vi "Usage3.vi"() -> ()   [LabVIEW 2017]
uses:
  Consumer/Abstract Consumer/Abstract Consumer.lvclass
  Message Queue/Message Queue/Message Queue.lvclass
  Message/Shutdown Message/Shutdown Message.lvclass
  SLSC Switch Consumer/SLSC Switch Consumer.lvclass
  Switch/Abstract Switch Init Parameters/Abstract Switch Init Parameters.lvclass
  Switch/Switch Connect Message/Switch Connect Message.lvclass
  Switch/Switch Disconnect All Message/Switch Disconnect All Message.lvclass
  Switch/Switch Disconnect Message/Switch Disconnect Message.lvclass
  Producer/Abstract Producer/Abstract Producer.lvclass
  Parameters/Abstract Init Parameters/Abstract Init Parameters.lvclass
  C:/azdo/jscholtz-message-queue-library/Source/Message Queue/Abstract Message Queue/Abstract Message Queue.lvclass
  C:/azdo/jscholtz-message-queue-library/Source/Switch/Abstract Switch Consumer/Abstract Switch Consumer.lvclass
  C:/azdo/jscholtz-message-queue-library/Source/Consumer/Abstract Consumer/Abstract Consumer.lvclass
  C:/azdo/jscholtz-message-queue-library/Source/Parameters/Abstract Init Parameters/Abstract Init Parameters.lvclass
  C:/azdo/jscholtz-message-queue-library/Source/Message/Abstract Request Message/Abstract Request Message.lvclass
  C:/azdo/jscholtz-message-queue-library/Source/Message/Abstract Message/Abstract Message.lvclass
panel:
  in  "Disconnect":bool
  in  "Disconnect All":bool
  in  "Connect":bool
  in  "Shutdown":bool
  out "error out":errorcluster
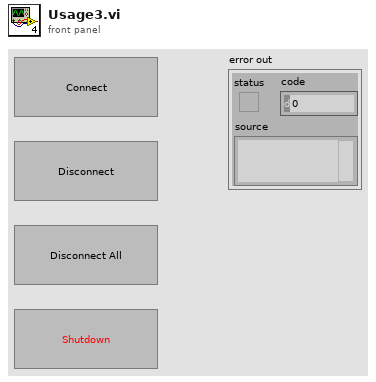
[diagram p1: front panel]
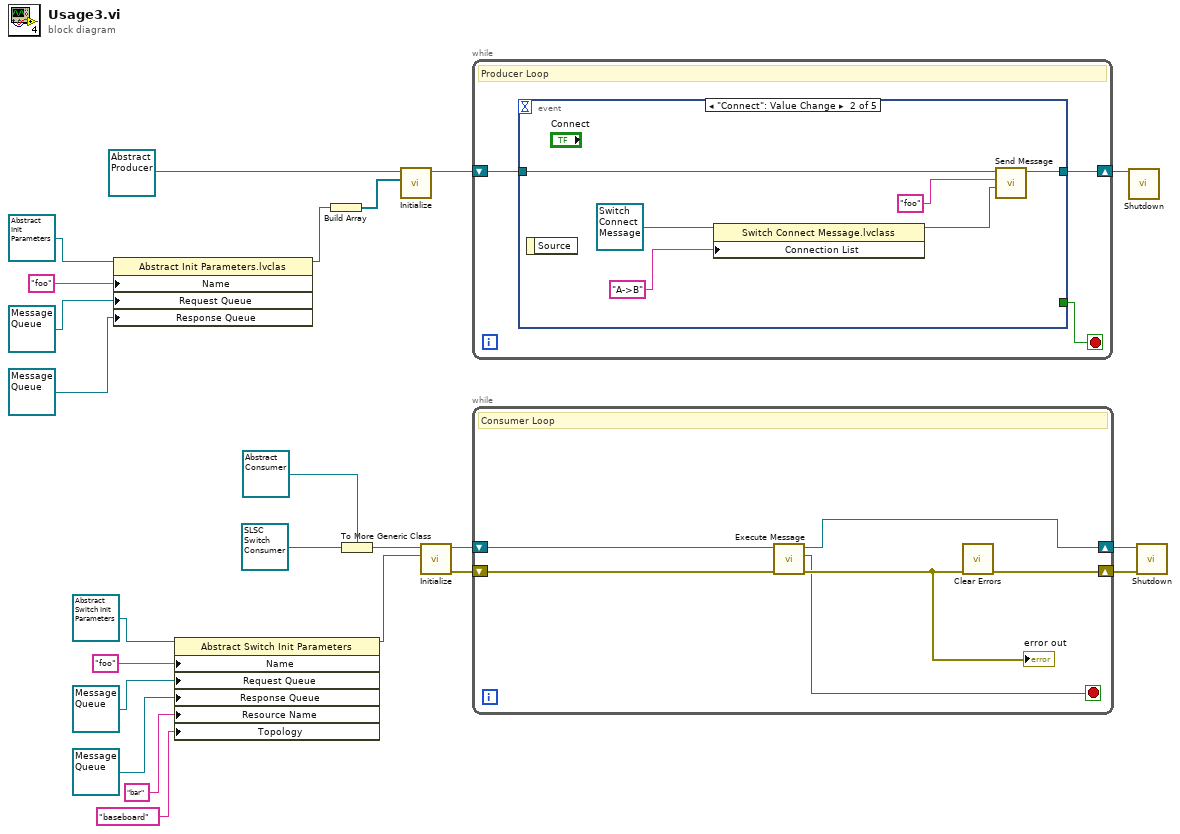
[diagram p0: block diagram]
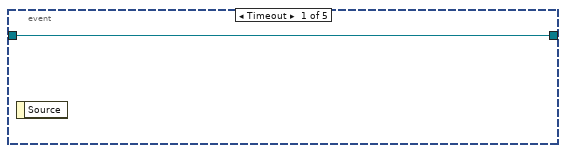
[diagram p2: hidden frame]
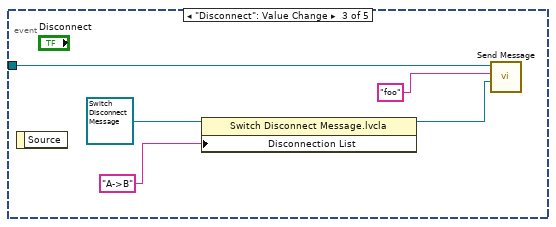
[diagram p3: hidden frame]
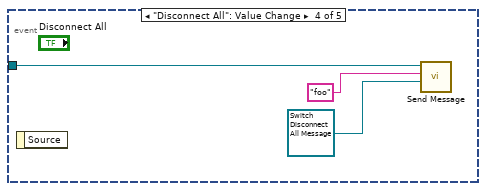
[diagram p4: hidden frame]
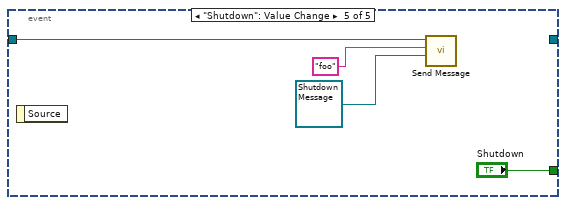
[diagram p5: hidden frame]
diagram:
  n1 = property class="Abstract Init Parameters.lvclas"(reference=refnum<class "Abstract Init Parameters.lvclass"> refnum ("Message Queue Library.lvlib:Abstract Init Parameters.lvclass"), "Name"="foo", "Request Queue"=refnum<class "Message Queue.lvclass"> refnum ("Message Queue Library.lvlib:Message Queue.lvclass"), "Response Queue"=refnum<class "Message Queue.lvclass"> refnum ("Message Queue Library.lvlib:Message Queue.lvclass")) -> (reference out=w3:refnum<class "Abstract Init Parameters.lvclass">)  [unwired: 1 in, 1 out]
  n2 = property class="Abstract Switch Init Parameters"(reference=refnum<class "Abstract Switch Init Parameters.lvclass"> refnum ("Message Queue Library.lvlib:Abstract Switch Init Parameters.lvclass"), "Name"="foo", "Request Queue"=refnum<class "Message Queue.lvclass"> refnum ("Message Queue Library.lvlib:Message Queue.lvclass"), "Response Queue"=refnum<class "Message Queue.lvclass"> refnum ("Message Queue Library.lvlib:Message Queue.lvclass"), "Resource Name"="bar", "Topology"="baseboard") -> (reference out=w18:refnum<class "Abstract Switch Init Parameters.lvclass">)  [unwired: 1 in, 1 out]
  n3 = Build Array(w3) -> (w8:refnum<class "Abstract Init Parameters.lvclass">[])
  n4 = To More Generic Class(target class=refnum<class "Abstract Consumer.lvclass"> refnum ("Abstract Consumer in"), reference=refnum<class "SLSC Switch Consumer.lvclass"> refnum ("Message Queue Library.lvlib:SLSC Switch Consumer.lvclass")) -> (generic class reference=w10:refnum<class "Abstract Consumer.lvclass">)
  n5 = call-dynamic "Initialize.vi"("Parameters in"=w8, "Abstract Producer in"=refnum<class "Abstract Producer.lvclass"> refnum ("Message Queue Library.lvlib:Abstract Producer.lvclass")) -> ("Abstract Producer out"=w2:refnum<class "Abstract Producer.lvclass">)  [unwired: 8 in, 1 out]
  n6 = call-dynamic "Initialize.vi"("Parameters in"=w18, "Abstract Consumer in"=w10) -> ("error out"=w23:errorcluster, "Abstract Consumer out"=w17:refnum<class "Abstract Consumer.lvclass">)  [unwired: 8 in]
  n7 = while {
    shift-right: [w24] -> w1
    shift-left: w2 -> [w25]
    stop <- w26 stop-if-true
    # "Producer Loop"
    n8 = event shown="[1] \"Connect\": Value Change" {
      selector: _ -> [_ _ _ _ _]
      dyn-events: _ -> [_ _ _ _ _]
      timeout: _ -> [_ _ _ _ _]
      tunnel: [_ _ _ _ "Shutdown"] -> w26
      tunnel: w25 -> [w27 w31 w35 w40 w43]
      tunnel: [w27 w28 _ _ _] -> w24
      event Timeout {
        n9 = event-data() -> ()  [unwired: 1 in, 1 out]
      }
      event "Connect": Value Change {
        n10 = event-data() -> ()  [unwired: 1 in, 1 out]
        n11 = property class="Switch Connect Message.lvclass"(reference=refnum<class "Switch Connect Message.lvclass"> refnum ("Message Queue Library.lvlib:Switch Connect Message.lvclass"), "Connection List"="A->B") -> (reference out=w30:refnum<class "Switch Connect Message.lvclass">)  [unwired: 1 in, 1 out]
        n12 = call-dynamic "Send Message.vi"("Message in"=w30, "Consumer in"="foo" ("Name"), "Abstract Producer in"=w31) -> ("Abstract Producer out"=w28:refnum<class "Abstract Producer.lvclass">)  [unwired: 6 in, 2 out]
      }
      event "Disconnect": Value Change {
        n13 = event-data() -> ()  [unwired: 1 in, 1 out]
        n14 = property class="Switch Disconnect Message.lvcla"(reference=refnum<class "Switch Disconnect Message.lvclass"> refnum ("Message Queue Library.lvlib:Switch Disconnect Message.lvclass"), "Disconnection List"="A->B" ("Connection List")) -> (reference out=w34:refnum<class "Switch Disconnect Message.lvclass">)  [unwired: 1 in, 1 out]
        n15 = call-dynamic "Send Message.vi"("Message in"=w34, "Consumer in"="foo" ("Name"), "Abstract Producer in"=w35) -> ()  [unwired: 6 in, 3 out]
      }
      event "Disconnect All": Value Change {
        n16 = event-data() -> ()  [unwired: 1 in, 1 out]
        n17 = call-dynamic "Send Message.vi"("Message in"=refnum<class "Switch Disconnect All Message.lvclass"> refnum ("Message Queue Library.lvlib:Switch Disconnect All Message.lvclass"), "Consumer in"="foo" ("Name"), "Abstract Producer in"=w40) -> ()  [unwired: 6 in, 3 out]
      }
      event "Shutdown": Value Change {
        n18 = event-data() -> ()  [unwired: 1 in, 1 out]
        n19 = call-dynamic "Send Message.vi"("Message in"=refnum<class "Shutdown Message.lvclass"> refnum ("Message Queue Library.lvlib:Shutdown Message.lvclass"), "Consumer in"="foo" ("Name"), "Abstract Producer in"=w43) -> ()  [unwired: 6 in, 3 out]
      }
    }
  }
  n20 = while {
    shift-right: [w46] -> w14
    shift-left: w23 -> [w51]
    shift-right: [w47] -> w13
    shift-left: w17 -> [w48]
    stop <- w49 stop-if-true
    # "Consumer Loop"
    n21 = call "Execute Message.vi"("error in (no error)"=w51, "Abstract Consumer in"=w48) -> ("error out"=w50:errorcluster, "Stop?"=w49:bool, "Abstract Consumer out"=w47:refnum<class "Abstract Consumer.lvclass">)  [unwired: 7 in]
    "error out" <- w50
    n22 = call <vilib>:"Clear Errors.vi"("error in (no error)"=w50) -> ("error out"=w46:errorcluster)  [unwired: 5 in, 1 out]
  }
  n23 = call-dynamic "Shutdown.vi"("Abstract Producer in"=w1) -> ()  [unwired: 9 in, 2 out]
  n24 = call-dynamic "Shutdown.vi"("error in (no error)"=w14, "Abstract Consumer in"=w13) -> ()  [unwired: 8 in, 2 out]
